vi "11_LAYOUT_COVID_19_ENUM.vi"() -> ()   [LabVIEW 2019]
panel:
  in  "Tab Control 2":enum32{"Page 1", "Page 2"}(ring)
  out "Numeric":i32
  in  "Tab Control":enum32{"Page 1", "Page 2"}(tab)
  out "Boolean":bool
  out "Boolean 2":bool
  in  "vi path":path
  in  "stop":bool
  # "LAYOUT --> TAB/SUB"
  # "SELECTOR TAB"
  # "(C) 2020"
  # "J.LUIS PÉREZ DEL VAL"
  # "GIF ANIMADO"
  # "KIT o CALENDARIO?..."
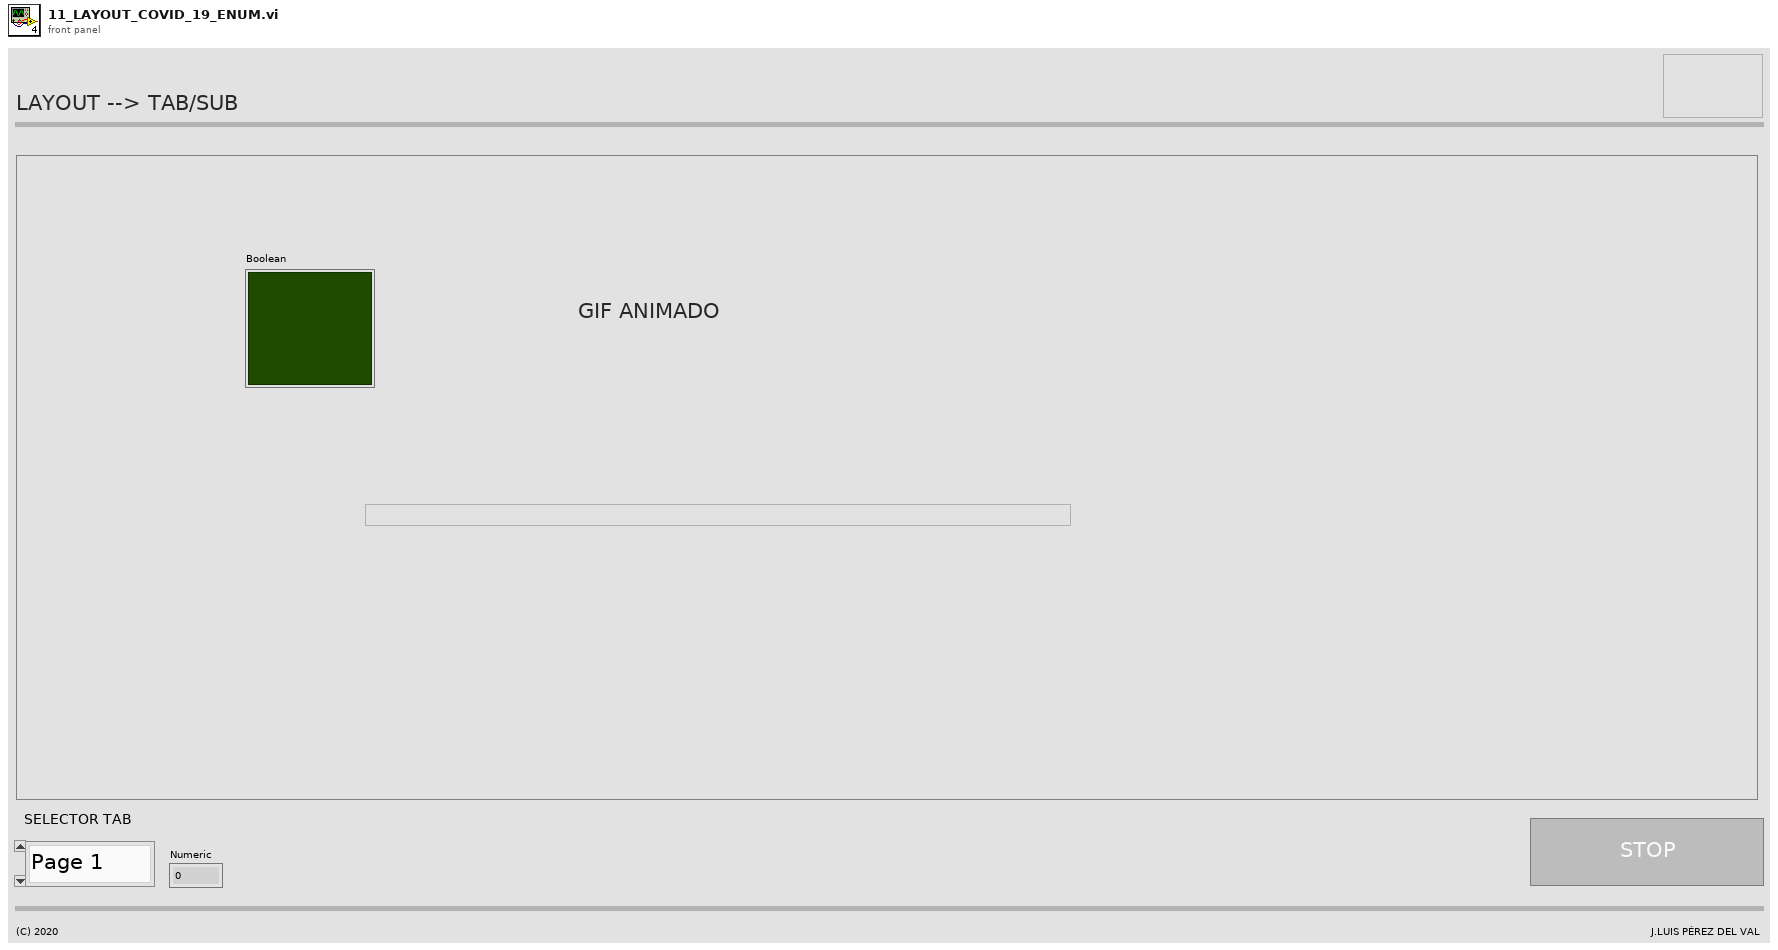
[diagram p1: front panel]
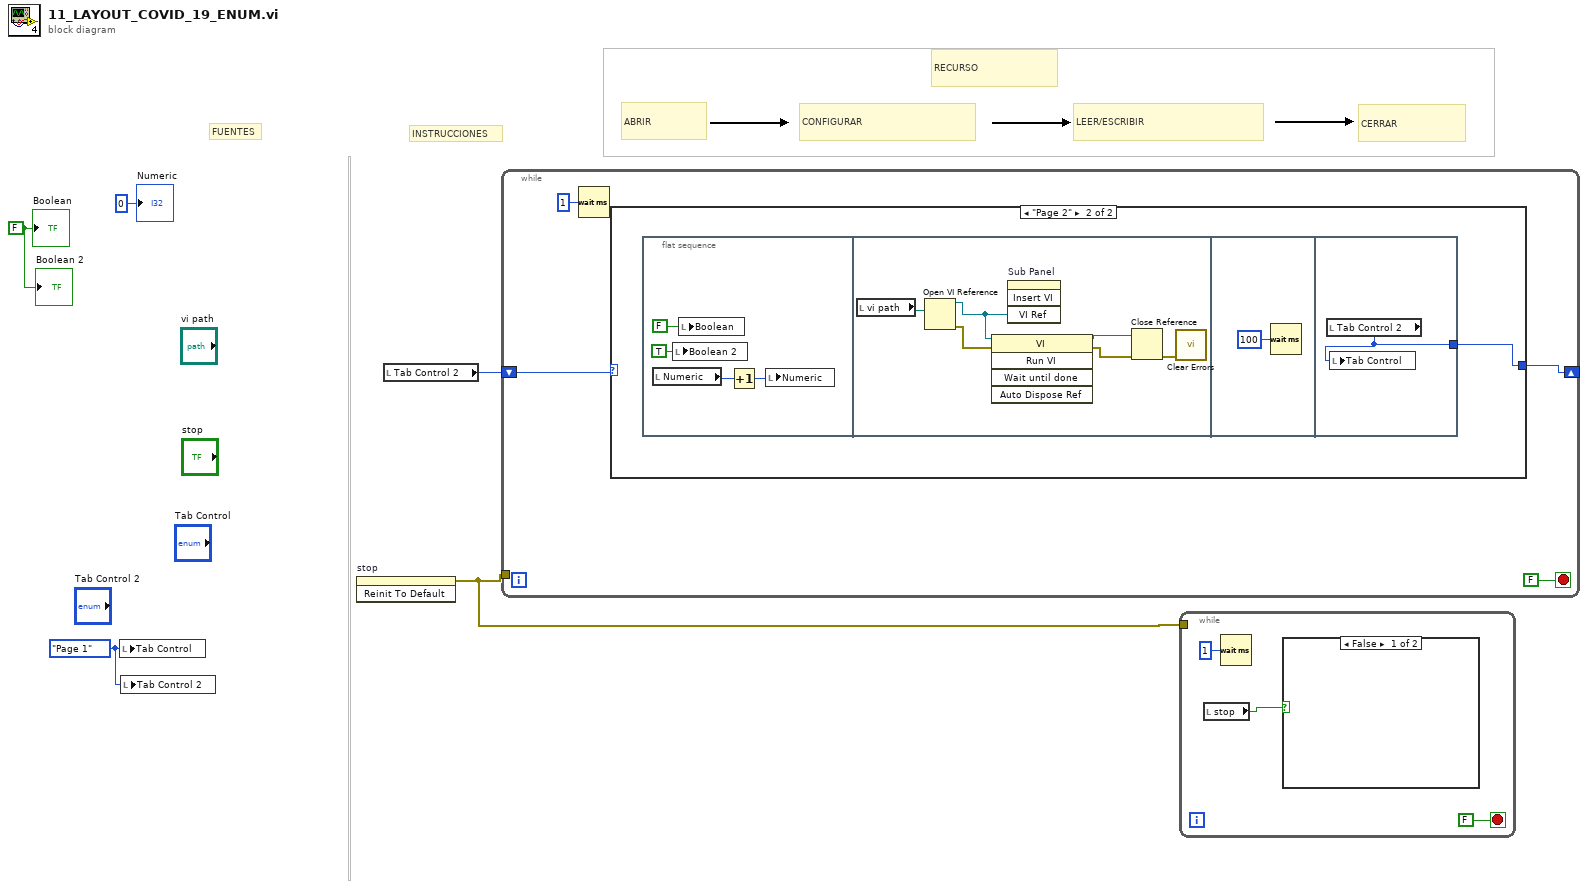
[diagram p0: block diagram]
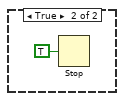
[diagram p2: hidden frame]
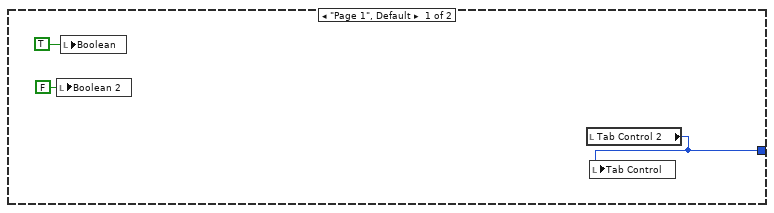
[diagram p3: hidden frame]
diagram:
  w1 = enum32{"Page 1", "Page 2"}."Page 1" ("Tab Control")
  w4 = FALSE ("Boolean")
  # "RECURSO"
  # "CERRAR"
  # "LEER/ESCRIBIR"
  # "CONFIGURAR"
  # "ABRIR"
  # "INSTRUCCIONES"
  # "FUENTES"
  n1 = local write "Tab Control"(w1) -> ()
  n2 = local write "Tab Control 2"(w1) -> ()
  n3 = invoke on="stop" class="Bool (strict)" method="Reinit To Default"() -> (error out=w5:errorcluster)  [unwired: 3 in, 2 out]
  n4 = local read "Tab Control 2"() -> (w2:enum32{"Page 1", "Page 2"})
  n5 = while {
    tunnel: w5 -> [_]
    shift-right: [w6] -> _
    shift-left: w2 -> [w7]
    stop <- FALSE stop-if-true
    n6 = Wait (ms)(milliseconds to wait=u32 1) -> ()  [unwired: 1 out]
    n7 = case shown="\"Page 2\"" w7 {
      tunnel: [w10 w13] -> w6
      frame "Page 1", Default {
        n8 = local write "Boolean 2"(FALSE ("INT_TAB")) -> ()
        n9 = local write "Boolean"(TRUE ("INT_TAB")) -> ()
        n10 = local read "Tab Control 2"() -> (w10:enum32{"Page 1", "Page 2"})
        n11 = local write "Tab Control"(w10) -> ()
      }
      frame "Page 2" {
        n12 = flat-sequence {
          tunnel: [w25] -> w13
          frame #0 {
            n13 = local read "Numeric"() -> (w15:i32)
            n14 = local write "Boolean 2"(TRUE ("INT_TAB")) -> ()
            n15 = local write "Boolean"(FALSE ("INT_TAB")) -> ()
            n16 = Increment(x=w15) -> (x+1=w14:i32)
            n17 = local write "Numeric"(w14) -> ()
          }
          frame #1 {
            n18 = local read "vi path"() -> (w21:path)
            n19 = Open VI Reference(vi path=w21) -> (vi reference=w20:refnum<vi>, error out=w19:errorcluster)  [unwired: 5 in]
            n20 = invoke class="VI" method="Run VI"(reference=w20, error in=w19) -> (reference out=w22:refnum<vi>, error out=w23:errorcluster)  [unwired: 3 in, 3 out]
            n21 = invoke on="Sub Panel" class="SubPnl" method="Insert VI"("VI Ref"=w20) -> ()  [unwired: 3 in, 4 out]
            n22 = Close Reference(reference=w22, error in (no error)=w23) -> (error out=w18:errorcluster)
            n23 = call <vilib>:"Clear Errors.vi"("error in (no error)"=w18) -> ()  [unwired: 5 in, 2 out]
          }
          frame #2 {
            n24 = Wait (ms)(milliseconds to wait=u32 100) -> ()  [unwired: 1 out]
          }
          frame #3 {
            n25 = local read "Tab Control 2"() -> (w25:enum32{"Page 1", "Page 2"})
            n26 = local write "Tab Control"(w25) -> ()
          }
        }
      }
    }
  }
  n27 = while {
    tunnel: w5 -> [_]
    stop <- FALSE stop-if-true
    n28 = local read "stop"() -> (w26:bool)
    n29 = Wait (ms)(milliseconds to wait=u32 1) -> ()  [unwired: 1 out]
    n30 = case shown="False" w26 {
      frame False {
      }
      frame True {
        n31 = Stop(stop? (T)=TRUE) -> ()
      }
    }
  }
  "Boolean" <- w4
  "Boolean 2" <- w4
  "Numeric" <- 0 ("Numeric")
